vi "actions整体图.vi"() -> ()   [LabVIEW 2014]
panel:
  in  "Cancel":bool
  in  "Apply":bool
  in  "Accept":bool
  in  "Warning":bool
  in  "Stop":bool
  in  "Ok":bool
  in  "No":bool
  in  "Important":bool
  in  "Exit":bool
  in  "Error":bool
  in  "Critical":bool
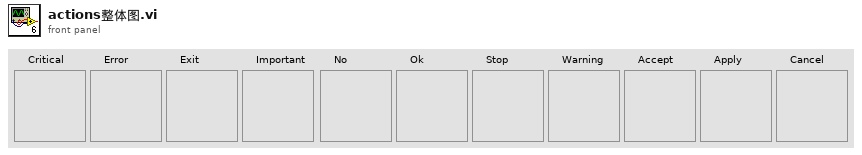
[diagram p1: front panel]
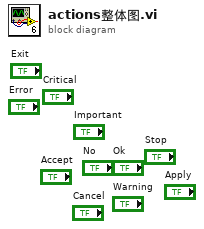
[diagram p0: block diagram]
diagram:
